vi "Corr Transducers File Dialog.vi"(8 "error in":errorcluster, 10 "channel index (0)":i32, 11 "transducers in":cluster{"channels":T1[], "last path":path} {"channels"."Phase index" min=1 step=1}) -> (0 "error out":errorcluster, 3 "transducers out":cluster{"channels":T1[], "last path":path} {"channels"."Phase index" min=1 step=1})   [LabVIEW 2013]
doc: "Shows file dialog for loading transducer file. If transducer is selected its path will be placed to the channels list or a new channel will be created in the list. But it does not load the file! It just sets its path."
uses:
  Corr Tranducer Item.ctl
panel:
  # "ADC:"
  # "ADC:"
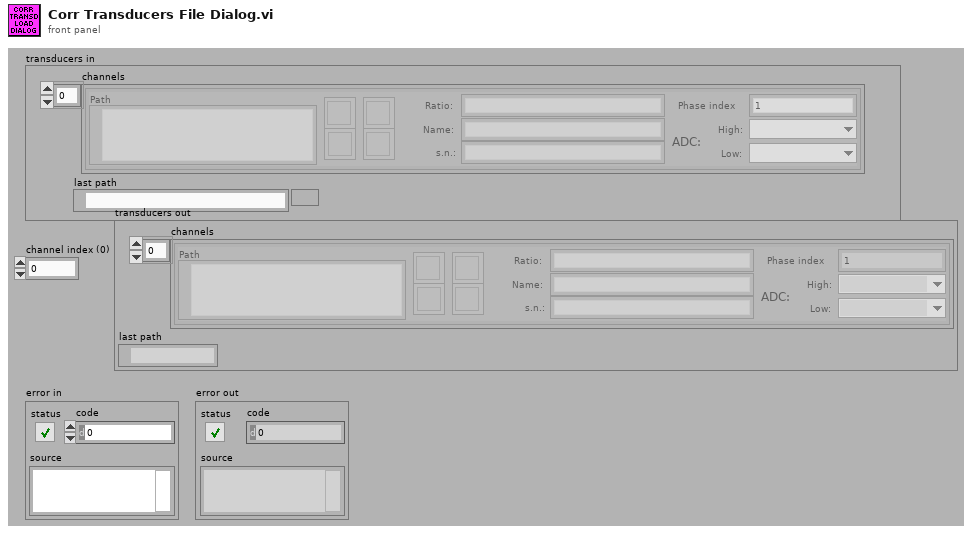
[diagram p1: front panel]
types:
  T1 = typedef "Corr Tranducer Item.ctl" = cluster{"Path":path, "Ratio:":string, "Name:":string, "btn rem":bool, "btn up":bool, "btn down":bool, "s.n.:":string, "btn open":bool, "ratio o/i":dbl, "chn hi":u16, "chn lo":u16, "Phase index":i32}
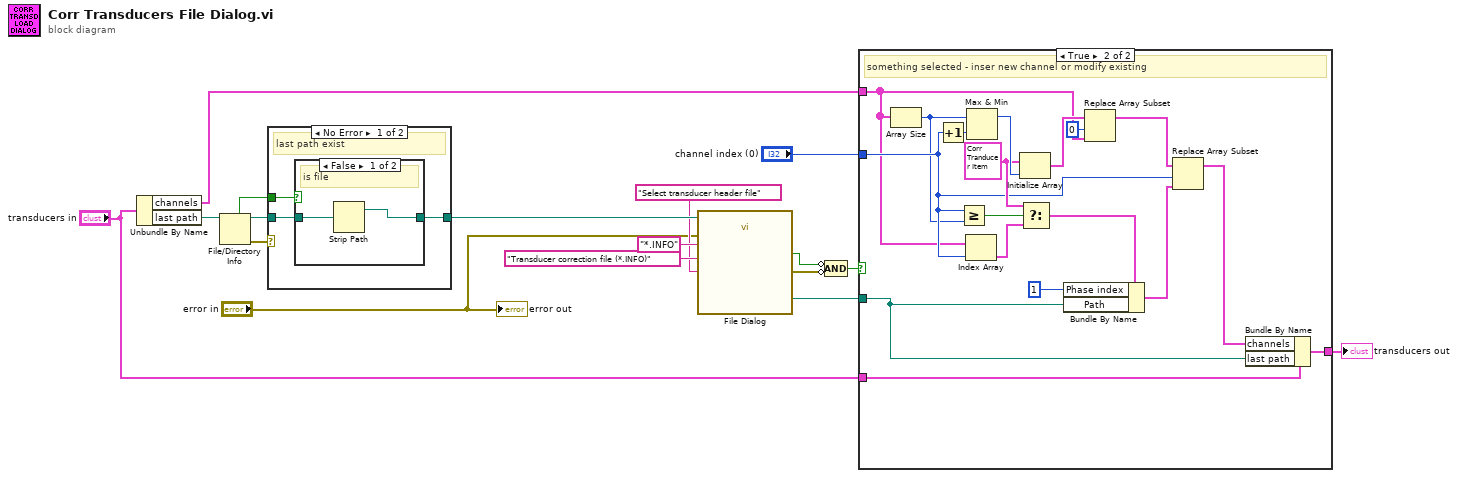
[diagram p0: block diagram]
diagram:
  n1 = Unbundle By Name("transducers in") -> ("channels"=w3:T1[], "last path"=w17:path)
  n2 = File/Directory Info(path=w17) -> (path out=w15:path, directory=w14:bool, error out=w16:errorcluster)  [unwired: 1 in, 4 out]
  n3 = case shown="No Error" w16 {
    tunnel: w15 -> [w19 w24]
    tunnel: w14 -> [w20 _]
    tunnel: [w18 w24] -> w13
    frame No Error {
      # "last path exist"
      n4 = case shown="False" w20 {
        tunnel: w19 -> [w22 w23]
        tunnel: [w21 w23] -> w18
        frame False {
          # "is file"
          n5 = Strip Path(path=w22) -> (stripped path=w21:path)  [unwired: 1 out]
        }
        frame True {
          # "is folder"
        }
      }
    }
    frame Error {
    }
  }
  n6 = call "File Dialog"("start path"=w13, "prompt"="Select transducer header file", "error in"="error in", "pattern (all files)"="*.INFO", "pattern label"="Transducer correction file (*.INFO)") -> ("selected path"=w6:path, "cancelled"=w9:bool, "error out"=w7:errorcluster)  [unwired: 7 in, 1 out]
  n7 = Compound Arithmetic op=AND(invert w9, invert w7) -> (w8:bool)
  n8 = case shown="True" w8 {
    tunnel: w6 -> [_ w34]
    tunnel: "transducers in" -> [w25 w43]
    tunnel: "channel index (0)" -> [_ w36]
    tunnel: w3 -> [_ w29]
    tunnel: [w25 w32] -> w1
    frame False {
    }
    frame True {
      w40 = T1 {"Path"=path "", "Ratio:"="", "Name:"="", "btn rem"=FALSE, "btn up"=FALSE, "btn down"=FALSE, "s.n.:"="", "btn open"=FALSE, "ratio o/i"=0.0, "chn hi"=0, "chn lo"=0, "Phase index"=0} ("Cluster")
      # "something selected - inser new channel or modify existing"
      n9 = Array Size(array=w29) -> (size(s)=w28:i32)
      n10 = Increment(x=w36) -> (x+1=w31:i32)
      n11 = Greater Or Equal?(x=w36, y=w28) -> (x >= y?=w41:bool)
      n12 = Index Array(array=w29, index=w36) -> (element=w39:T1)
      n13 = Max & Min(x=w28, y=w31) -> (max(x,y)=w42:i32)  [unwired: 1 out]
      n14 = Initialize Array(w40, w42) -> (w30:T1[])
      n15 = Select(t=w40, s=w41, f=w39) -> (s? t:f=w38:T1)
      n16 = Bundle By Name(cluster=w38, "Phase index"=1, "Path"=w34) -> (w37:T1)
      n17 = Replace Array Subset(array=w30, new element=w29, index=0) -> (w27:T1[])
      n18 = Replace Array Subset(array=w27, new element=w37, index=w36) -> (w33:T1[])
      n19 = Bundle By Name(cluster=w43, "channels"=w33, "last path"=w34) -> (w32:cluster{"channels":T1[], "last path":path})
    }
  }
  "transducers out" <- w1
  "error out" <- "error in"
